vi "formula note.vi"() -> ()   [LabVIEW 2020]
panel:
  in  "B":dbl
  in  "A":dbl
  out "C":dbl
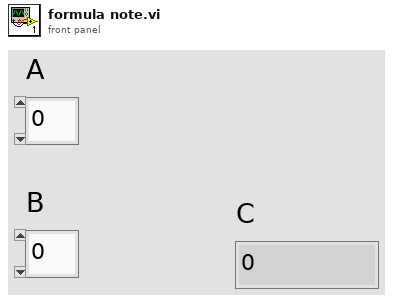
[diagram p1: front panel]
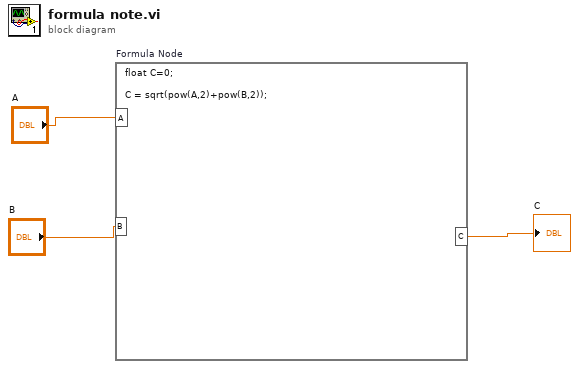
[diagram p0: block diagram]
diagram:
  n1 = formula code="float C=0;\n\nC = sqrt(pow(A,2)+pow(B,2));"("A"="A", "B"="B") -> ("C"=→"C":dbl)
